vi "Sine Scale.vi"(2 "bypass":bool, 3 "Amplify":dbl(knob)=4.036434060236755 scale=0.0..10.0, 4 "Sensor":dbl, 5 "Input":dbl) -> (1 "Output":dbl)   [LabVIEW 2012]
panel:
  in  "90 Deg Offset":dbl=67.5
  # "Maximum force on Elevator Motor\nis when linkage is at 90 deg, which is\nwhen Shooter is at 22.5 deg\n90 - 22.5 = 67.5 deg offset"
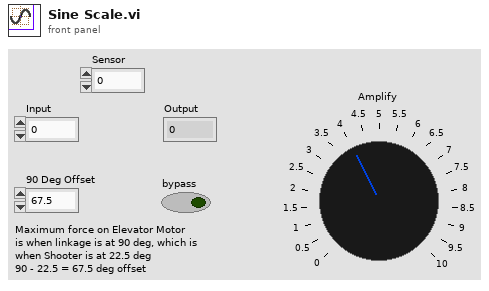
[diagram p1: front panel]
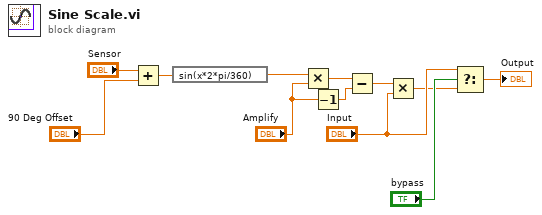
[diagram p0: block diagram]
diagram:
  n1 = Add(x="Sensor", y="90 Deg Offset") -> (x+y=w11:dbl)
  n2 = expression code="sin(x*2*pi/360)"(w11) -> (w10:dbl)
  n3 = Multiply(x=w10, y="Amplify") -> (x*y=w9:dbl)
  n4 = Decrement(x="Amplify") -> (x-1=w6:dbl)
  n5 = Subtract(x=w9, y=w6) -> (x-y=w7:dbl)
  n6 = Multiply(x=w7, y="Input") -> (x*y=w2:dbl)
  n7 = Select(t="Input", s="bypass", f=w2) -> (s? t:f=→"Output":dbl)
